vi "Test Process Error Handler Configured.vi"(8 "error in (no error)":errorcluster, 11 "Process Test In":refnum<class "Process Test.lvclass">) -> (0 "error out":errorcluster, 3 "Process Test Out":refnum<class "Process Test.lvclass">)   [LabVIEW 2020, in "Process Test.lvclass"]
uses:
  Process Test.lvclass
  C:/Program Files (x86)/National Instruments/LabVIEW 2020/vi.lib/Astemes/LUnit/Test Case.lvclass
  Mock Error Handler/Mock Error Handler.lvclass
  C:/Git/astemes-triarc-framework/source/Framework/Error Handler Interface/Error Handler Interface.lvclass
  Framework/Process/Process.lvclass/Process.ctl
  <vilib>/Astemes/LUnit/Test Case.lvclass/Test Case.ctl
  <vilib>/Astemes/LUnit/LUnit Assertion Result.lvclass/LUnit Assertion Result.ctl
  <vilib>/Astemes/LUnit/LUnit Test Case Result.lvclass/LUnit Test Case Result.ctl
  <vilib>/Astemes/LUnit/LUnit Method Result.lvclass/LUnit Method Result.ctl
  Framework/Process/Protected/Messaging/Send Message.vi
  Framework/Process/Public/Lifecycle/Get Lifecycle State.vi
  <vilib>/Astemes/LUnit/Palette/Fail.vi
  <vilib>/Astemes/LUnit/Palette/Pass.vi
  <vilib>/Astemes/LUnit/Set Assertion Type.vi
  Framework/Process/Private/SubVIs/Handle Debug Data.vi
  <vilib>/Utility/error.llb/Clear Errors.vi
  <vilib>/Astemes/LUnit/Add test result.vi
  <vilib>/Astemes/LUnit/LUnit Write Passed.vi
  <vilib>/Astemes/LUnit/LUnit Write Message.vi
  <vilib>/Astemes/LUnit/LUnit Write Description.vi
  <vilib>/Astemes/LUnit/LUnit Write Assertion Type.vi
  Framework/Logging/Log Debug.vi
  <vilib>/AdvancedString/1D String Array to Delimited String.vi
  <vilib>/Utility/High Resolution Relative Seconds.vi
  <vilib>/Astemes/LUnit/LUnit Record Assertion Result.vi
  <vilib>/Astemes/LUnit/LUnit Aggregate Assertion Results.vi
  <vilib>/Astemes/LUnit/Assertion Result/LUnit Read Status.vi
  <vilib>/Astemes/LUnit/LUnit Read Message.vi
  <vilib>/Astemes/LUnit/LUnit Read Description.vi
  <vilib>/Astemes/LUnit/Method Result/LUnit Merge Status.vi
  <vilib>/Astemes/LUnit/LUnit Concatenate result strings.vi
  <vilib>/Utility/error.llb/Error Cluster From Error Code.vi
  Framework/Process/Public/Read Name.vi
  <vilib>/Astemes/LUnit/LUnit Assertion Result.lvclass
  Framework/Process/Process.lvclass
  Process Test.lvclass/Process Test.ctl
  <vilib>/Astemes/LUnit/Test Case.lvclass
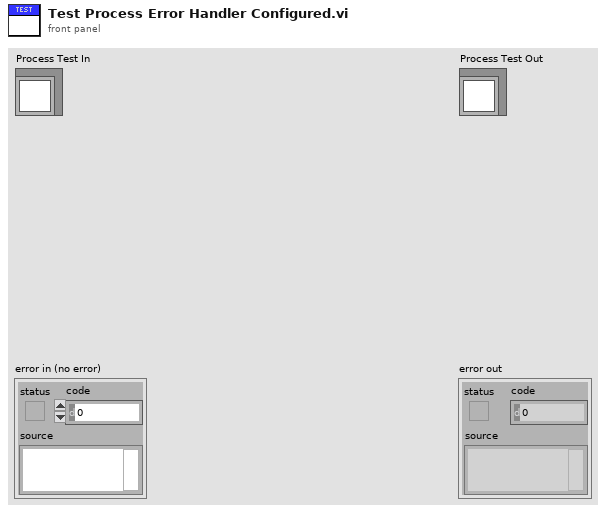
[diagram p1: front panel]
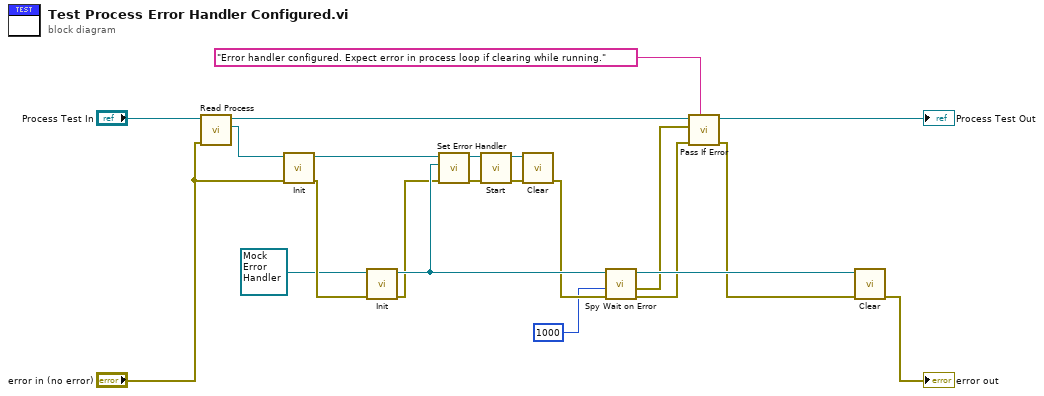
[diagram p0: block diagram]
diagram:
  n1 = call "Read Process.vi"("error in (no error)"="error in (no error)", "Process Test in"="Process Test In") -> ("Process.lvclass"=w10:refnum<class "Process.lvclass">, "Process Test out"=w9:refnum<class "Process Test.lvclass">)  [unwired: 7 in, 1 out]
  n2 = call-dynamic "Init.vi"("error in (no error)"="error in (no error)", "Process In"=w10) -> ("error out"=w21:errorcluster, "Process Out"=w4:refnum<class "Process.lvclass">)  [unwired: 8 in]
  n3 = call-dynamic "Init.vi"("error in (no error)"=w21, "Mock Error Handler In"=refnum<class "Mock Error Handler.lvclass"> refnum ("Mock Error Handler.lvclass")) -> ("error out"=w5:errorcluster, "Mock Error Handler Out"=w18:refnum<class "Mock Error Handler.lvclass">)  [unwired: 8 in]
  n4 = call "Set Error Handler.vi"("error in (no error)"=w5, "Error Handler"=w18, "Process In"=w4) -> ("error out"=w19:errorcluster, "Process Out"=w2:refnum<class "Process.lvclass">)  [unwired: 7 in]
  n5 = call "Start.vi"("error in (no error)"=w19, "Process In"=w2) -> ("error out"=w3:errorcluster, "Process Out"=w1:refnum<class "Process.lvclass">)  [unwired: 7 in, 1 out]
  n6 = call-dynamic "Clear.vi"("error in (no error)"=w3, "Process In"=w1) -> ("error out"=w15:errorcluster)  [unwired: 9 in]
  n7 = call "Spy Wait on Error.vi"("error in (no error)"=w15, "timeout in ms (-1)"=1000, "Mock Error Handler In"=w18) -> ("error out"=w14:errorcluster, "Errors"=w13:errorcluster, "Mock Error Handler Out"=w17:refnum<class "Mock Error Handler.lvclass">)  [unwired: 4 in, 2 out]
  n8 = call <vilib>:"Pass If Error.vi"("Description"="Error handler configured. Expect error in process loop if clearing while running.", "error in (no error)"=w14, "Assert error"=w13, "LUnit Test Case In"=w9) -> ("error out"=w12:errorcluster, "LUnit Test Case Out"=→"Process Test Out":refnum<class "Process Test.lvclass">)  [unwired: 6 in]
  n9 = call-dynamic "Clear.vi"("error in (no error)"=w12, "Mock Process In"=w17) -> ("error out"=→"error out":errorcluster)  [unwired: 9 in]
